vi "Reference Precision Type.vi"(10 "error in (no error)":errorcluster) -> (2 "error out":errorcluster, 3 "Precision Type":refnum<vi>)   [LabVIEW 2018, in "Numeric Data Type.lvclass"]
uses:
  Numeric Data Type.lvclass
  Precision Type.ctl
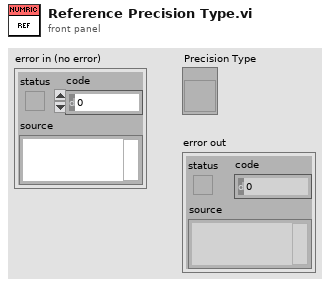
[diagram p1: front panel]
types:
  T1 = typedef "Numeric Data Type.lvclass/UI References.ctl" = cluster{"Main Tab":refnum<vi>, "Column Header":refnum<vi>, "Default Value":refnum<vi>, "Default Value (Complex)":refnum<vi>, "Default Value (Date/Time)":refnum<vi>, "Representation":refnum<vi>, "Fixed-Point Configuration":refnum<vi>, "Use Default Limits":refnum<vi>, "Limits Mode Tab":refnum<vi>, "Minimum":refnum<vi>, "Maximum":refnum<vi>, "Increment":refnum<vi>, "Minimum Time":refnum<vi>, "Maximum Time":refnum<vi>, "Coerce Minimum":refnum<vi>, "Coerce Maximum":refnum<vi>, "Coerce Increment":refnum<vi>, "Min/Max Warning":refnum<vi>, "Editing Mode":refnum<vi>, "Default/Advanced Tab":refnum<vi>, "Time/Numeric Tab":refnum<vi>, "Display Type":refnum<vi>, "Digits":refnum<vi>, "Precision Type":refnum<vi>, "Hide Zeros":refnum<vi>, "Exponent":refnum<vi>, "Use Min Width":refnum<vi>, "Min Field Width":refnum<vi>, "Padding":refnum<vi>, "Time Format":refnum<vi>, "Clock Type":refnum<vi>, "Include Seconds":refnum<vi>, "HMS Digits":refnum<vi>, "Date Format":refnum<vi>, "Date Order":refnum<vi>, "Year Format":refnum<vi>, "Format String":refnum<vi>, "Valid":refnum<vi>, "Revert":refnum<vi>, "List Type":refnum<vi>, "Format Codes":refnum<vi>, "Insert":refnum<vi>}
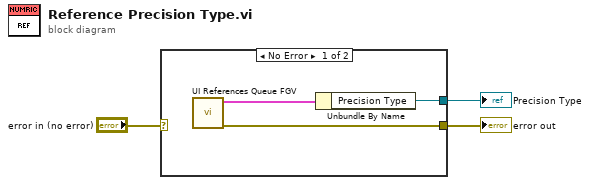
[diagram p0: block diagram]
diagram:
  n1 = case shown="No Error" "error in (no error)" {
    selector: "error in (no error)" -> [_ w7]
    tunnel: [w4 w7] -> w2
    tunnel: [w5 _] -> w1
    frame No Error {
      n2 = call "UI References Queue FGV.vi"() -> ("error out"=w4:errorcluster, "UI References out"=w6:T1)  [unwired: 10 in]
      n3 = Unbundle By Name(w6) -> ("Precision Type"=w5:refnum<vi>)
    }
    frame Error {
    }
  }
  "error out" <- w2
  "Precision Type" <- w1
